vi "Generate State Information.vi"(8 "error in (no error)":errorcluster, 11 "Abstract Routing Channel Template in":refnum<class "Abstract Routing Channel Template.lvclass">) -> (0 "error out":errorcluster, 2 "State Configurations":T1[](array[typedef])=[{"Name"="No Connections", "Description"="State with no connections", "Value"=-1, "Connection List"=[]}], 3 "Abstract Routing Channel Template out":refnum<class "Abstract Routing Channel Template.lvclass">)   [LabVIEW 2020, in "Routing Templates.lvlib" / "Abstract Routing Channel Template.lvclass"]
uses:
  Abstract Routing Channel Template.lvclass
  Abstract Routing Channel Template.lvclass/Abstract Routing Channel Template.ctl
  Shared/Connection.ctl
  Shared/Routing and Faulting Shared.lvlib
  Shared/Routing State.ctl
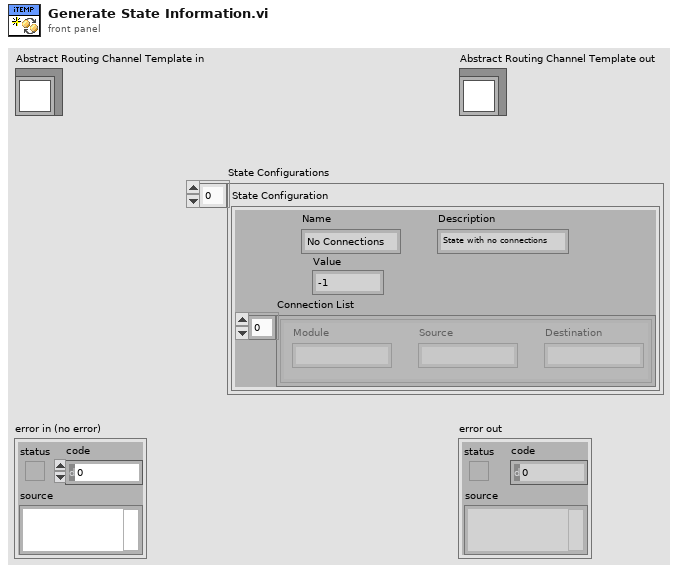
[diagram p1: front panel]
types:
  T1 = typedef "Routing and Faulting Shared.lvlib/Routing State.ctl" = cluster{"Name":string, "Description":string, "Value":i32, "Connection List":T2[]}
  T2 = typedef "Routing and Faulting Shared.lvlib/Connection.ctl" = cluster{"Module":string, "Source":string, "Destination":string}
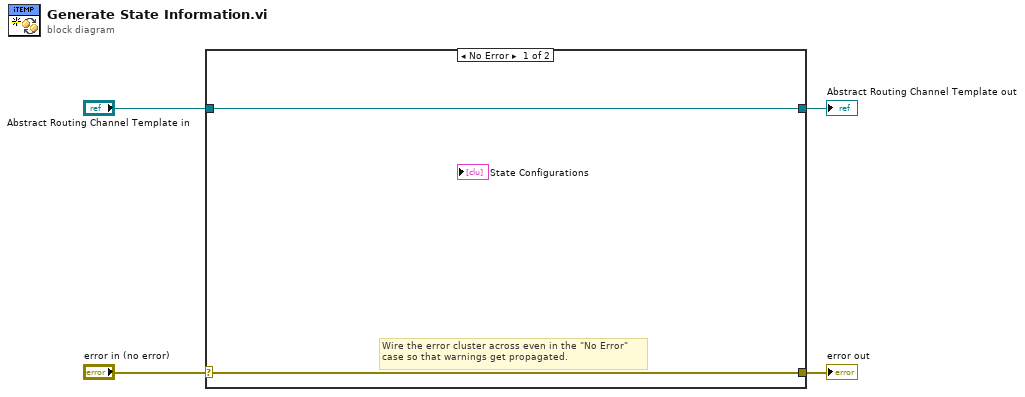
[diagram p0: block diagram]
diagram:
  n1 = case shown="No Error" "error in (no error)" {
    selector: "error in (no error)" -> [w5 w8]
    tunnel: [w5 w8] -> w3
    tunnel: [w6 w7] -> w1
    tunnel: "Abstract Routing Channel Template in" -> [w6 w7]
    frame No Error {
      # "Wire the error cluster across even in the \"No Error\"\ncase so that warnings get propagated."
    }
    frame Error {
    }
  }
  "error out" <- w3
  "Abstract Routing Channel Template out" <- w1
